vi "Test Base Card Passthrough (Relay).vi"() -> ()   [LabVIEW 2020, in "slsc-switch-benchmarks.lvlib"]
uses:
  slsc-switch-benchmarks.lvlib
panel:
  out "error out":errorcluster
  in  "Disconnection":enum16{"Open All", "Disconnect All"}(ring)=enum."Disconnect All"
  in  "Iterations":u32=1000
  in  "Channels to Sweep":i32=64
  out "#Channels Testing":i32
  out "Avg Connection Time":dbl(graph)
  in  "device":refnum<k21>="SET-2010-Mod2"
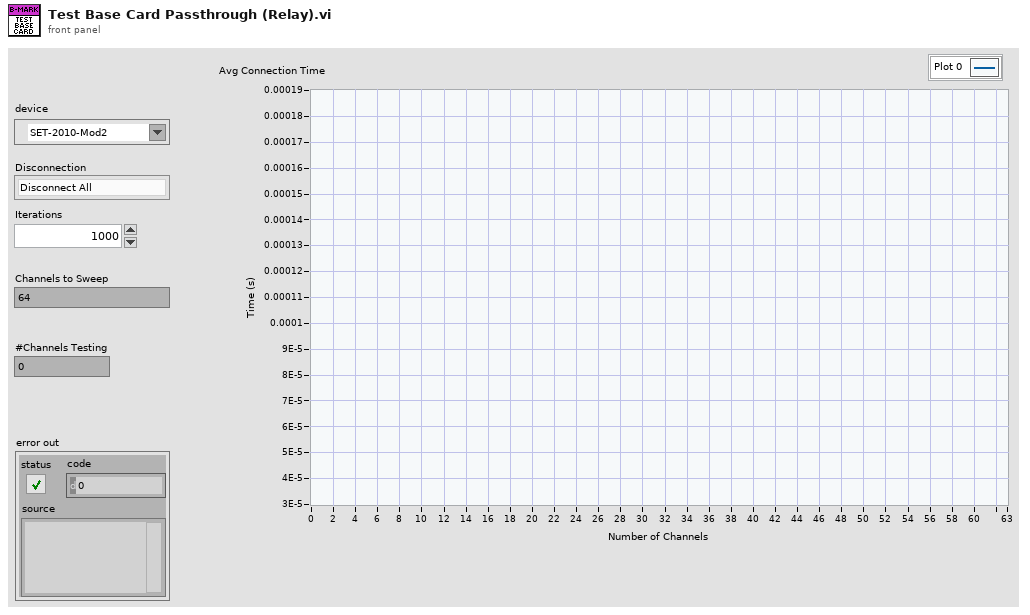
[diagram p1: front panel]
types:
  T1 = typedef "slsc-switch-benchmarks.lvlib/Timing Statistics.ctl" = cluster{"mean":dbl, "standard deviation":dbl, "maximum time":dbl, "minimum time":dbl}
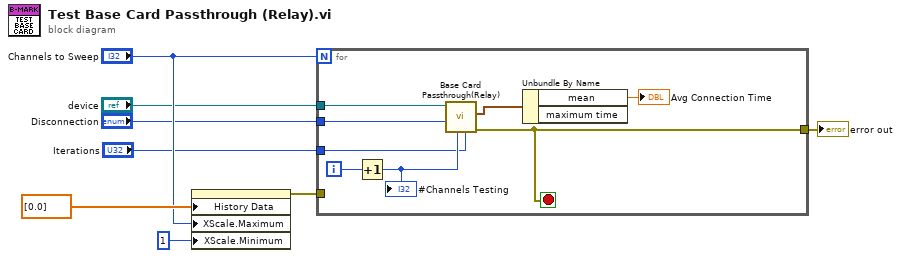
[diagram p0: block diagram]
diagram:
  n1 = property on="Avg Connection Time" class="WFChart (strict)"("History Data"=dbl[] [0.0], "XScale.Maximum"="Channels to Sweep", "XScale.Minimum"=1 ("Channels to Sweep")) -> (error out=w7:errorcluster)  [unwired: 2 in, 1 out]
  n2 = for {
    N: "Channels to Sweep" -> [_]
    tunnel: "device" -> [w15]
    tunnel: w7 -> [_]
    tunnel: "Iterations" -> [w12]
    tunnel: "Disconnection" -> [w11]
    tunnel: [w10] -> w2
    i -> [w16]
    stop <- w10 stop-if-true
    n3 = Increment(x=w16) -> (x+1=w13:i32)
    "#Channels Testing" <- w13
    n4 = call "Base Card Passthrough(Relay).vi"("Iterations"=w12, "Channels (1-64)"=w13, "Disconnection"=w11, "device"=w15) -> ("error out"=w10:errorcluster, "Connect Timing"=w14:T1)  [unwired: 5 in, 1 out]
    n5 = Unbundle By Name(w14) -> ("mean"=→"Avg Connection Time":dbl)  [unwired: 1 out]
  }
  "error out" <- w2
